vi "SetMoveTolerance.vi"() -> (2 "Max Pulses":u32)   [LabVIEW 2015]
uses:
  Anemometry/Anemometry Sub Vis/Globals/Constants_global.vi
  Anemometry/Anemometry Sub Vis/Globals/Trav_pos_global.vi
  <vilib>/Utility/config.llb/Read Key (U32).vi
  <vilib>/Utility/config.llb/Write Key (U32).vi
  <vilib>/Utility/config.llb/NI_LVConfig.lvlib
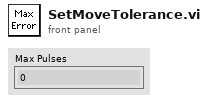
[diagram p1: front panel]
types:
  T1 = typedef "NI_LVConfig.lvlib/Config Data RefNum.ctl" = refnum<k1>
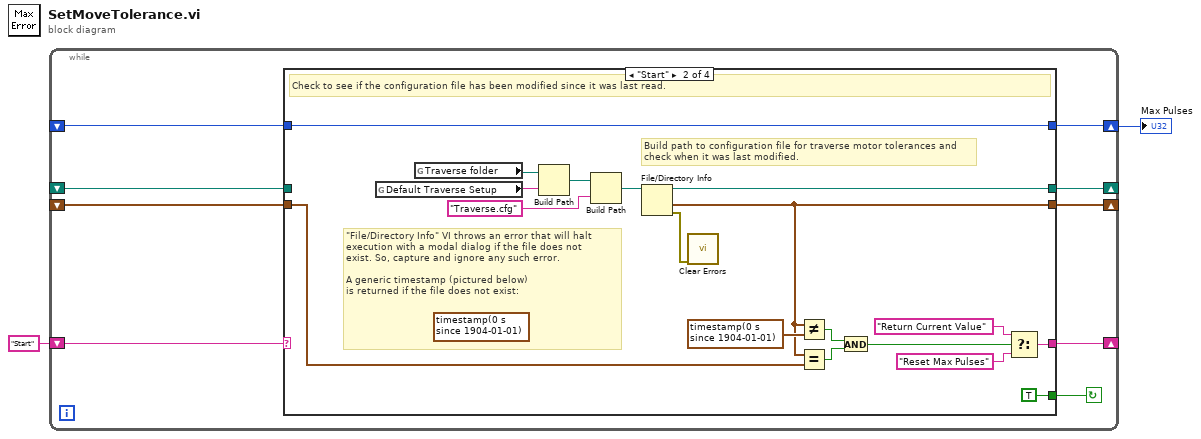
[diagram p0: block diagram]
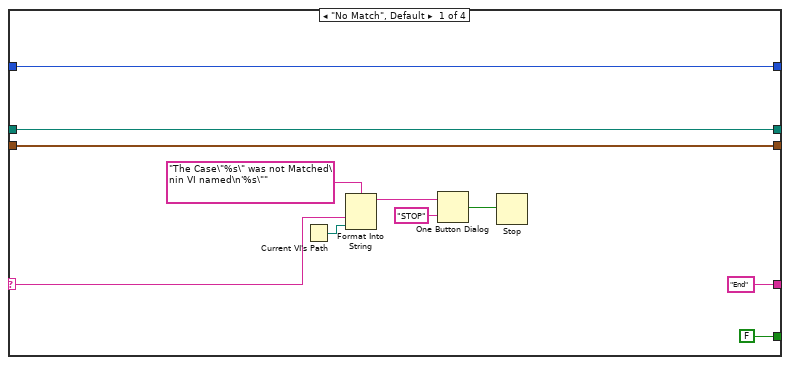
[diagram p2: hidden frame]
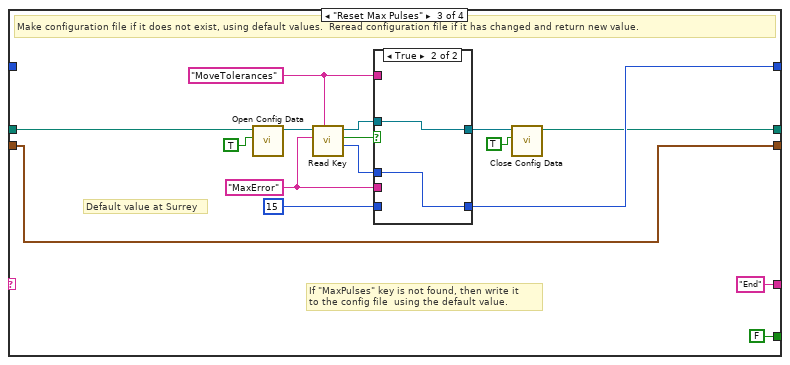
[diagram p3: hidden frame]
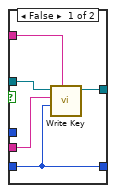
[diagram p4: hidden frame]
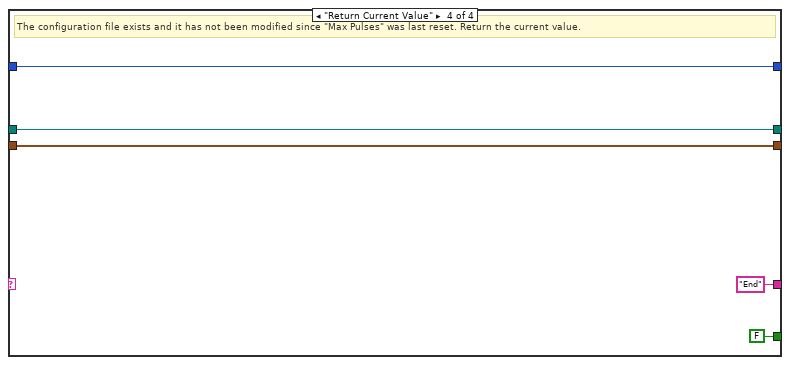
[diagram p5: hidden frame]
diagram:
  n1 = while {
    shift-left: _ -> [w5]
    shift-right: [w7] -> _
    shift-left: _ -> [w6]
    shift-right: [w8] -> w1
    shift-left: "Start" -> [w9]
    shift-right: [w10] -> _
    shift-right: [w4] -> _
    shift-left: _ -> [w3]
    stop <- w11 continue-if-true
    n2 = case shown="\"Start\"" w9 {
      selector: w9 -> [w13 _ _ _]
      tunnel: [FALSE TRUE FALSE FALSE] -> w11
      tunnel: ["End" w31 "End" "End"] -> w10
      tunnel: [w15 w34 w45 w68] -> w8
      tunnel: [w14 w28 w42 w67] -> w7
      tunnel: w6 -> [w15 w34 _ w68]
      tunnel: w5 -> [w14 w30 w42 w67]
      tunnel: [w12 w23 w43 w64] -> w4
      tunnel: w3 -> [w12 _ w44 w64]
      frame "No Match", Default {
        n3 = Current VI's Path() -> (path=w17:path)
        n4 = Format Into String(format string="The Case\"%s\" was not Matched\nin VI named\n'%s\"" ("Format String"), w13, w17) -> (resulting string=w20:string)  [unwired: 2 in, 1 out]
        n5 = One Button Dialog(message=w20, button name ("OK")="STOP") -> (true=w18:bool)
        n6 = Stop(stop? (T)=w18) -> ()
      }
      frame "Start" {
        (unwired) timestamp(0 s since 1904-01-01) ("last mod")
        # "Build path to configuration file for traverse motor tolerances and check when it was last modified."
        # "Check to see if the configuration file has been modified since it was last read."
        # "\"File/Directory Info\" VI throws an error that will halt execution with a modal dialog if the file does not \nexist. So, capture and ignore any such error.\n\nA generic timestamp (pictured below) is returned if the file does not exist:"
        # "\"File/Directory Info\" VI throws an error that will halt execution with a modal dialog if the file does not \nexist. So, capture and ignore any such error.\n\nA generic timestamp (pictured below)\nis returned if the file does not exist:"
        # "\"File/Directory Info\" VI throws an error that will halt execution with a modal dialog if the file does not \nexist. So, capture and ignore any such error.\n\nA generic timestamp (pictured below)\nis returned if the file does not exist:"
        n7 = global read "Trav_pos_global.vi" "Default Traverse Setup"() -> (w40:string)
        n8 = global read "Constants_global.vi" "Traverse folder"() -> (w39:path)
        n9 = Build Path(base path=w39, name or relative path=w40) -> (appended path=w37:path)
        n10 = Build Path(base path=w37, name or relative path="Traverse.cfg") -> (appended path=w36:path)
        n11 = File/Directory Info(path=w36) -> (path out=w23:path, last mod=w28:timestamp, error out=w35:errorcluster)  [unwired: 1 in, 4 out]
        n12 = call <vilib>:"Clear Errors.vi"("error in (no error)"=w35) -> ()  [unwired: 5 in, 2 out]
        n13 = Not Equal?(x=w28, y=timestamp(0 s since 1904-01-01) ("last mod")) -> (x != y?=w27:bool)
        n14 = Equal?(x=w28, y=w30) -> (x = y?=w26:bool)
        n15 = And(x=w27, y=w26) -> (x .and. y?=w32:bool)
        n16 = Select(t="Return Current Value", s=w32, f="Reset Max Pulses") -> (s? t:f=w31:string)
      }
      frame "Reset Max Pulses" {
        w52 = "MoveTolerances" ("section")
        w51 = "MaxError" ("key")
        # "If \"MaxPulses\" key is not found, then write it\nto the config file  using the default value."
        # "Default value at Surrey"
        # "Make configuration file if it does not exist, using default values.  Reread configuration file if it has changed and return new value."
        n17 = call <vilib>:"Open Config Data.vi"("create file if necessary (T)"=TRUE, "configuration file path"=w44) -> ("refnum"=w48:T1)  [unwired: 7 in, 2 out]
        n18 = call-poly <vilib>:"Read Key.vi"("section"=w52, "key"=w51, "refnum"=w48) -> ("value"=w50:u32, "found?"=w49:bool, "refnum out"=w54:T1)  [unwired: 5 in, 1 out]
        n19 = case shown="True" w49 {
          tunnel: w50 -> [_ w63]
          tunnel: w51 -> [w59 _]
          tunnel: w52 -> [w60 _]
          tunnel: u32 15 ("value") -> [w58 _]
          tunnel: [w58 w63] -> w45
          tunnel: w54 -> [w61 w62]
          tunnel: [w57 w62] -> w46
          frame False {
            n20 = call-poly <vilib>:"Write Key.vi"("section"=w60, "value"=w58, "key"=w59, "refnum"=w61) -> ("refnum out"=w57:T1)  [unwired: 5 in, 2 out]
          }
          frame True {
          }
        }
        n21 = call <vilib>:"Close Config Data.vi"("write file if changed (T)"=TRUE, "refnum"=w46) -> ("file path"=w43:path)  [unwired: 8 in, 1 out]
      }
      frame "Return Current Value" {
        # "The configuration file exists and it has not been modified since \"Max Pulses\" was last reset. Return the current value."
      }
    }
  }
  "Max Pulses" <- w1
